vi "DAC V vs freq sweep with leveling.vi"() -> ()   [LabVIEW 2012]
uses:
  <vilib>/Analysis/1siggen.llb/Ramp Pattern by Samples.vi
  <vilib>/Utility/file.llb/Write To Spreadsheet File (DBL).vi
  <vilib>/express/express arith-compare/Formula/XNode/ExpressFormulaBlockNode.xnode
  <vilib>/Analysis/NI_AALBase.lvlib
panel:
  in  "leveling file":path=path "C:/Users/Ouyang Group/Documents/Data/8-5-16/wavetek power calibration double sweep -4dbm interp 3"
  in  "file path (dialog if empty)":path
  in  "resolution (1 Hz:1)":i32(ring)=1 items=["0.1 Hz", "1 Hz", "10 Hz", "100 Hz", "1 KHz", "10 KHz", "100 KHz", "1 MHz", "10 MHz", "100 MHz", "1 GHz"]
  in  "band (1-26.5 GHz:20)":i32(ring)=2
  in  "GPIB Address":string="19"
  in  "f start":dbl format="%0.2f"
  in  "f end":dbl=1.0 format="%0.2f"
  in  "f samples":i32=128
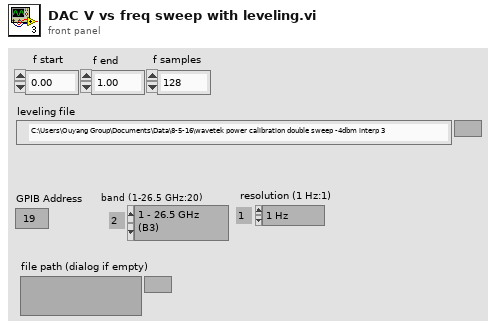
[diagram p1: front panel]
types:
  T1 = cluster{"power\nmeter":bool, bool, "Power Offset":ext}
  T2 = cluster{"source lock":bool, "lock frequency (Hz)":ext, "coarse tune":bool}
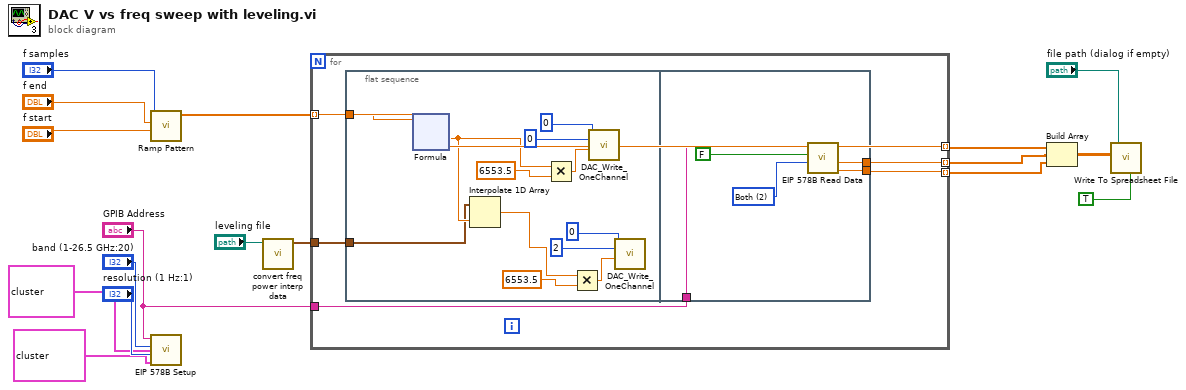
[diagram p0: block diagram]
diagram:
  n1 = call-poly <vilib>:"Ramp Pattern.vi"("start"="f start", "end"="f end", "samples"="f samples") -> ("Ramp Pattern"=w5:dbl[])  [unwired: 7 in, 1 out]
  n2 = call "EIP 578B Setup.vi"("GPIB Address"="GPIB Address", "band (1-26.5 GHz:20)"="band (1-26.5 GHz:20)", "resolution (1 Hz:1)"="resolution (1 Hz:1)", "source locking"=T2 {"source lock"=FALSE, "lock frequency (Hz)"=1000000000.0, "coarse tune"=FALSE}, "power meter"=T1 {"power\nmeter"=TRUE, FALSE, "Power Offset"=0.0}) -> ()  [unwired: 1 in, 2 out]
  n3 = call "convert freq power interp data.vi"("file path (dialog if empty)"="leveling file") -> ("Array"=w1:cluster{dbl, dbl}[])  [unwired: 10 in]
  n4 = for {
    tunnel: w5 -> [w20] mode=indexing
    tunnel: "GPIB Address" -> [w22]
    tunnel: [w21] -> w4 mode=indexing
    tunnel: [w20] -> w13 mode=indexing
    tunnel: [w19] -> w3 mode=indexing
    tunnel: w1 -> [w18]
    n5 = flat-sequence {
      tunnel: w20 -> [w24]
      tunnel: w18 -> [w23]
      tunnel: w22 -> [w45]
      tunnel: [w44] -> w21
      tunnel: [w43] -> w19
      frame #0 {
        n6 = xnode "Formula"("X1"=w24) -> ("Result"=w30:dbl)  [unwired: 1 in, 1 out]
        n7 = Interpolate 1D Array(1:w30, 2:w23) -> (0:w25:dbl)
        n8 = Multiply(x=w30, y=6553.5) -> (x*y=w33:dbl)
        n9 = Multiply(x=w25, y=6553.5) -> (x*y=w28:dbl)
        n10 = call "DAC_Write_OneChannel.vi"("Value"=w33, "Channel"=u16 0, "DeviceIndex"=u64 0) -> ()  [unwired: 7 in, 2 out]
        n11 = call "DAC_Write_OneChannel.vi"("Value"=w28, "Channel"=u16 2, "DeviceIndex"=u64 0) -> ()  [unwired: 7 in, 2 out]
      }
      frame #1 {
        w47 = 2 items=["Frequency", "Power", "Both"] ("output mode (freq:0)")
        n12 = call "EIP 578B Read Data.vi"("output mode (freq:0)"=w47, "fast (T=active)"=FALSE, "GPIB"=w45) -> ("Power (dBm)"=w43:ext, "frequency (Hz)"=w44:ext)  [unwired: 1 in, 2 out]
      }
    }
  }
  n13 = Build Array(w13, w4, w3) -> (w9:ext[][])
  n14 = call-poly <vilib>:"Write To Spreadsheet File.vi"("transpose? (no:F)"=TRUE, "2D data"=w9, "file path (dialog if empty)"="file path (dialog if empty)") -> ()  [unwired: 5 in, 1 out]
